vi "Invalid Ref.vi"(1 "PropertyObject":refnum<class "PropertyObject.lvclass">) -> (0 "Not a Valid Ref?":bool)   [LabVIEW 2020, in "TSnax.lvlib" / "PropertyObject.lvclass"]
uses:
  PropertyObject.lvclass
  PropertyObject.lvclass/PropertyObject.ctl
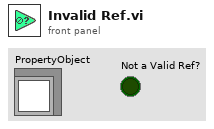
[diagram p1: front panel]
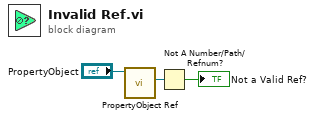
[diagram p0: block diagram]
diagram:
  n1 = call "PropertyObject Ref.vi"("PropertyObject in"="PropertyObject") -> ("PropertyObject"=w2:refnum<k7>)  [unwired: 8 in, 2 out]
  n2 = Not A Number/Path/Refnum?(number/path/refnum=w2) -> (NaN/Path/Refnum?=→"Not a Valid Ref?":bool)
